vi "TreeNode Get Descendants.vi"(8 "error in (no error)":errorcluster, 11 "TreeNode DVR in":refnum<data-value>) -> (0 "error out":errorcluster, 2 "TreeNodeArray":refnum<data-value>[](array[refnum]), 3 "TreeNode DVR out":refnum<data-value>)   [LabVIEW 2012, in "MDSplus.lvlib"]
uses:
  <vilib>/MDSplus/Library/MDSplus.lvlib
  <vilib>/MDSplus/Classes/Data_Class/TreeNode_Class/TreeNode.lvclass
panel:
  out "Descendants":i64[](array[numeric])
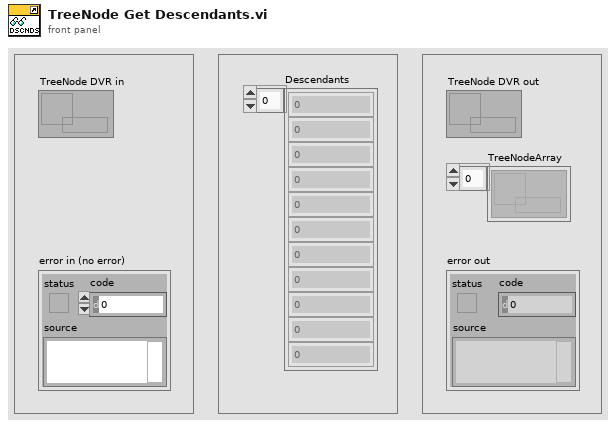
[diagram p1: front panel]
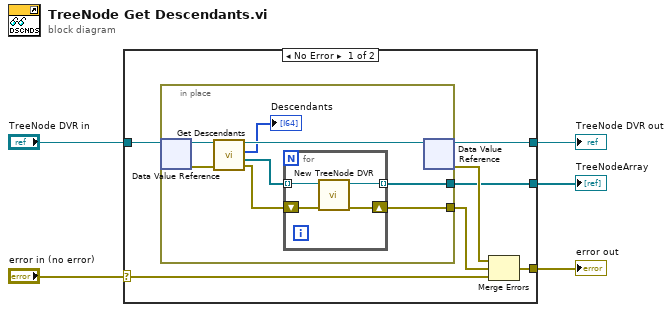
[diagram p0: block diagram]
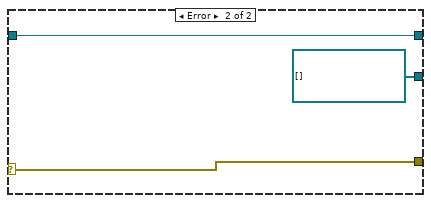
[diagram p2: hidden frame]
diagram:
  n1 = case shown="No Error" "error in (no error)" {
    selector: "error in (no error)" -> [w11 w27]
    tunnel: "TreeNode DVR in" -> [w12 w26]
    tunnel: [w8 w27] -> w5
    tunnel: [w9 w26] -> w2
    tunnel: [w6 refnum<data-value>[] []] -> w1
    frame No Error {
      n2 = in-place {
        in-place-border: [w13] -> w7
        in-place-border: [w16] -> w6
        n3 = in-place-dvr #1(w12) -> (w20:refnum<class "TreeNode.lvclass">, w19:errorcluster)
        n4 = call-dynamic "Get Descendants.vi"("error in (no error)"=w19, "TreeNode in"=w20) -> ("error out"=w14:errorcluster, "TreeNodeArray"=w17:refnum<class "TreeNode.lvclass">[], "Descendants"=→"Descendants":i64[], "TreeNode out"=w18:refnum<class "TreeNode.lvclass">)  [unwired: 6 in]
        n5 = for {
          tunnel: w17 -> [w24] mode=indexing
          tunnel: [w23] -> w16 mode=indexing
          shift-right: [w21] -> w13
          shift-left: w14 -> [w22]
          n6 = call <vilib>:"New TreeNode DVR.vi"("error in (no error)"=w22, "TreeNode in"=w24) -> ("error out"=w21:errorcluster, "TreeNode DVR out"=w23:refnum<data-value>)  [unwired: 8 in]
        }
        n7 = in-place-dvr #1(w18) -> (w9:refnum<data-value>, w10:errorcluster)
      }
      n8 = Merge Errors(w10, w7, w11) -> (w8:errorcluster)
    }
    frame Error {
    }
  }
  "error out" <- w5
  "TreeNode DVR out" <- w2
  "TreeNodeArray" <- w1
